vi "Template jsObject Array.vi"(8 "error in (no error)":errorcluster, 9 "TEMPLATES (none)":T1[](array[typedef]), 10 "Array Name (\"TEMPLATES\")":string="TEMPLATES", 11 "Previous String (\"\")":string) -> (0 "error out":errorcluster, 2 "Templates jsObject Array":string, 3 "Template jsObject Definition":string)   [LabVIEW 2011]
uses:
  Template Record.ctl
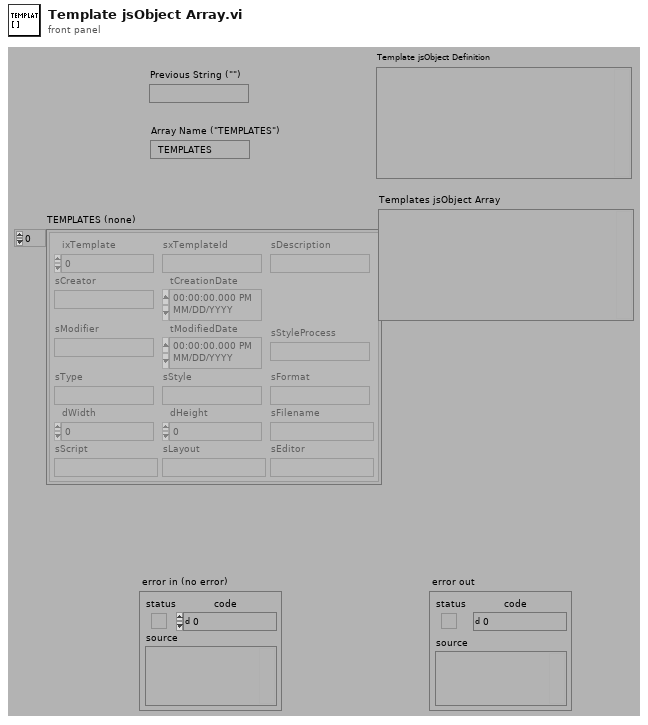
[diagram p1: front panel]
types:
  T1 = typedef "Template Record.ctl" = cluster{"ixTemplate":i32, "sxTemplateId":string, "sDescription":string, "sCreator":string, "tCreationDate":timestamp, "sModifier":string, "tModifiedDate":timestamp, "sType":string, "sStyle":string, "sFormat":string, "dWidth":dbl, "dHeight":dbl, "sFilename":string, "sScript":string, "sLayout":string, "sEditor":string, "sStyleProcess":string}
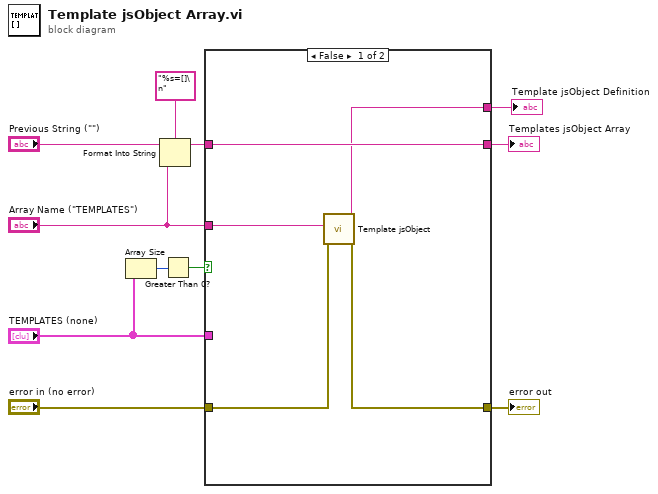
[diagram p0: block diagram]
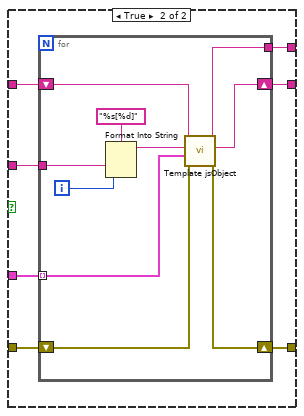
[diagram p2: hidden frame]
diagram:
  n1 = Array Size(array="TEMPLATES (none)") -> (size(s)=w3:i32)
  n2 = Format Into String(format string="%s=[]\n", initial string="Previous String (\"\")", "Array Name (\"TEMPLATES\")") -> (resulting string=w10:string)  [unwired: 1 in, 1 out]
  n3 = Greater Than 0?(x=w3) -> (x > 0?=w2:bool)
  n4 = case shown="False" w2 {
    tunnel: "TEMPLATES (none)" -> [_ w23]
    tunnel: w10 -> [w13 w22]
    tunnel: "error in (no error)" -> [w16 w21]
    tunnel: [w13 w20] -> w7
    tunnel: [w15 w19] -> w6
    tunnel: "Array Name (\"TEMPLATES\")" -> [w14 w18]
    tunnel: [w12 w17] -> w1
    frame False {
      n5 = call "Template jsObject.vi"("error in (no error)"=w16, "Template jsObject Name (\"\")"=w14) -> ("error out"=w15:errorcluster, "Template jsObject Definition"=w12:string)  [unwired: 2 in, 6 out]
    }
    frame True {
      n6 = for {
        tunnel: w23 -> [w32] mode=indexing
        shift-right: [w24] -> w20
        shift-left: w22 -> [w33]
        shift-right: [w30] -> w19
        shift-left: w21 -> [w31]
        tunnel: w18 -> [w26]
        tunnel: [w25] -> w17
        i -> [w27]
        n7 = Format Into String(format string="%s[%d]", w26, w27) -> (resulting string=w28:string)  [unwired: 2 in, 1 out]
        n8 = call "Template jsObject.vi"("error in (no error)"=w31, "Template Record (empty)"=w32, "Template jsObject Name (\"\")"=w28, "Previous String (\"\")"=w33) -> ("error out"=w30:errorcluster, "Template jsObject"=w24:string, "Template jsObject Definition"=w25:string)  [unwired: 5 out]
      }
    }
  }
  "Templates jsObject Array" <- w7
  "error out" <- w6
  "Template jsObject Definition" <- w1
